vi "TSLIN_SetData.vi"(8 "Error in":errorcluster caption="error in (no error)", 9 "AppName":string="LABFD", 10 "Set":T1={"Hardware Type"=3, "Hardware Subtype"=enum."TC1026", "AHwChannel"=0, "AAppChannel"=0, "ABaudrateKbps"=19.2, "AProtocol"=2, "AldHW"=0} {"Hardware Type" items=["BUS_UNKNOWN_TYPE", "TS_TCP_DEVICE", "XL_USB_DEVICE", "TS_USB_DEVICE", "PEAK_USB_DEVICE", "KVASER_USB_DEVICE", "ZLG_USB_DEVICE", "ICS_USB_DEVICE", "TS_TC1005_DEVICE", "CANABLE_USB_DEVICE", "TS_WIRELESS_OBD", "TS_USB_DEVICE_EX", "IXXAT_USB_DEVICE", "TS_ETH_IF_DEVICE", "TS_USB_IF_DEVICE", "BUS_DEV_TYPE_COUNT"]; "AHwChannel" items=["CHN1", "CHN2", "CHN3", "CHN4", "CHN5", "CHN6", "CHN7", "CHN8", "CHN9", "CHN10", "CHN11", "CHN12", "CHN13", "CHN14", "CHN15", "CHN16", "CHN17", "CHN18", "CHN19", "CHN20", "CHN21", "CHN22", "CHN23", "CHN24", "CHN25", "CHN26", "CHN27", "CHN28", "CHN29", "CHN30", "CHN31", "CHN32"]; "AAppChannel" items=["CHN1", "CHN2", "CHN3", "CHN4", "CHN5", "CHN6", "CHN7", "CHN8", "CHN9", "CHN10", "CHN11", "CHN12", "CHN13", "CHN14", "CHN15", "CHN16", "CHN17", "CHN18", "CHN19", "CHN20", "CHN21", "CHN22", "CHN23", "CHN24", "CHN25", "CHN26", "CHN27", "CHN28", "CHN29", "CHN30", "CHN31", "CHN32"]; "AProtocol" items=["Lin_Protocol_13", "Lin_Protocol_20", "Lin_Protocol_21", "Lin_Protocol_J2602"]}, 11 "Path":path) -> (0 "Error out":errorcluster caption="error out", 1 "mapping_return":i32, 2 "config_baud_return":i32, 3 "Path output":path)   [LabVIEW 2014]
doc: "tsapp_set_mapping_verbose ：\nFunction Introduction ：\nBefore using hardware devices, map the channels (CAN/CANFD/LIN) for the application program\n(i.e. binding) specifies the designated channel of the CAN device. This operation can also be performed on\nThe device management interface of TSMaster is completed, and this part of the operation is not required in the code.\nRegarding the channel mapping function, there are still unclear areas. Please refer to the document: TsMasterApi HardwareMap.pdf\nCall location ：\nCall this function to complete the hardware binding before the application connects to the CAN tool.\ninput parameter \nAppName: Application Name: The name of the application bound to this Map, which should be consistent with the name in initialized lib_tsmaster\nagreement\nAAppChannelType: Channel type: including APP_CAN, APP_LIN AAppChannel: Channel number of the application: This is the channel number used by the upper level program\nAHardwareName: Hardware name: such as TOSUN, Vector, etc., can also be left blank, mainly for the convenience of users to view\nAHardwareType: Hardware type: According to TLIBBusToolDeviceType, it includes all mainstream CANs currently on the market\nCard hardware Among them, the definition of tool enumeration types is as follows:\npublic enum TLIBBusToolDeviceType : int {\nBUS_UNKNOWN_TYPE = 0, TS_TCP_DEVICE = 1, XL_USB_DEVICE = 2, TS_USB_DEVICE = 3, PEAK_USB_DEVICE = 4, KVASER_USB_DEVICE = 5, ZLG_USB_DEVICE = 6, ICS_USB_DEVICE = 7, TS_TC1005_DEVICE = 8\n};\nAHardwareSubType: The sub devices under this device type, such as TS-USB-Device on the same star, are included below TC1001, TL1002, TC1011 and other series of products\nAHardwareIndex: Supports inserting multiple identical hardware devices simultaneously, such as inserting two TC1001 devices at the same time. This is used to select\nIs it the channel of device 1 or device 2\nAHardwareChannel: The channel for hardware devices, for example, TC1005 has 5 hardware channels, and this parameter is used to select the appropriate one\nCorresponding hardware channels\nAEnable Mapping: Is this mapping enabled? If set to false, the channel cannot be used。\nReturn value ：\n==0: Execution successful\nOther: Query error code\n\ntsapp_configure_baudrate_lin :\nFunction Introduction\nSet parameters such as baud rate for LIN channel\nCall location\nBefore connecting hardware devices, set the parameters of the channel first\ninput parameter \nAIdxChnq: Application Channel Number\nABaud rate Kbps: baud rate (kbps)\nAProtocol: baud rate (kbps)\nReturn value\n==0: Connection successful\nOther: Check for error codes"
uses:
  Typedef/TSLIN_SetData.ctl
  Utilities/Typedef/Hardware_Subtype.ctl
  All_Control/Typedef/Hardware Type.ctl
panel:
  # "Use N CAN channels and set N CAN channels"
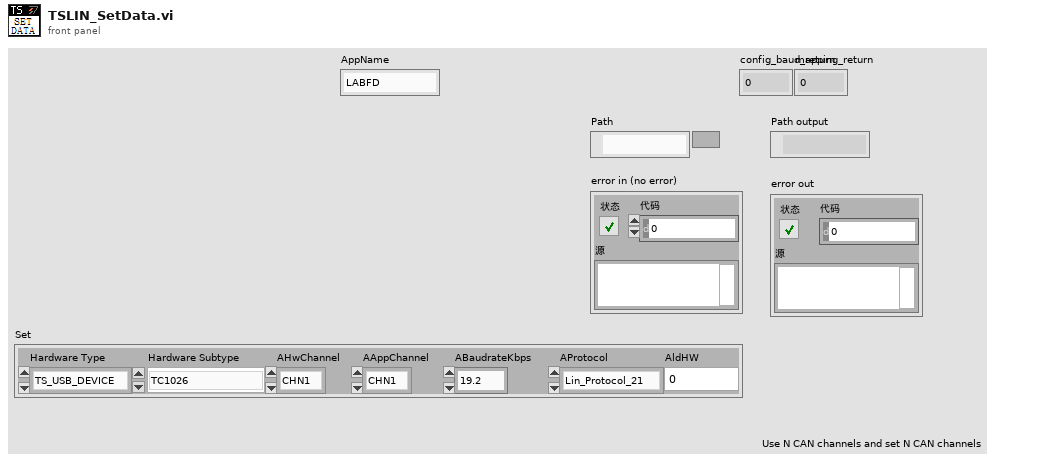
[diagram p1: front panel]
types:
  T1 = typedef "TSLIN_SetData.ctl" = cluster{"Hardware Type":T2, "Hardware Subtype":T3, "AHwChannel":i32, "AAppChannel":i32, "ABaudrateKbps":sgl, "AProtocol":i32, "AldHW":i32}
  T2 = typedef "Hardware Type.ctl" = i32
  T3 = typedef "Hardware_Subtype.ctl" = enum16{"TS_UNKNOWN_DEVICE", "TSCAN_PRO", "TSCAN_Lite1", "TC1001", "TL1001", "TC1011", "TM5011", "TC1002", "TC1014", "TSCANFD2517", "TC1026", "TC1016", "TC1012", "TC1013", "TLog1002", "TC1034", "TC1018", "GW2116", "TC2115", "MP1013", "TC1113", "TC1114", "TP1013", "TC1017", "TP1018", "TF10XX", "TL1004_FD_4_LIN_2", "TE1051", "TP1051", "TP1034", "TTS9015", "TP1026", "TTS1026", "TTS1034", "TTS1018", "TL1011", "TTS1015_LiAuto", "TTS1013_LiAuto", "TTS1016Pro", "TC1054Pro", "TC1054", "TLog1038", "TO1013", "TC1034Pro", "TC1018Pro", "TC1038Pro", "TS_DEV_END"}
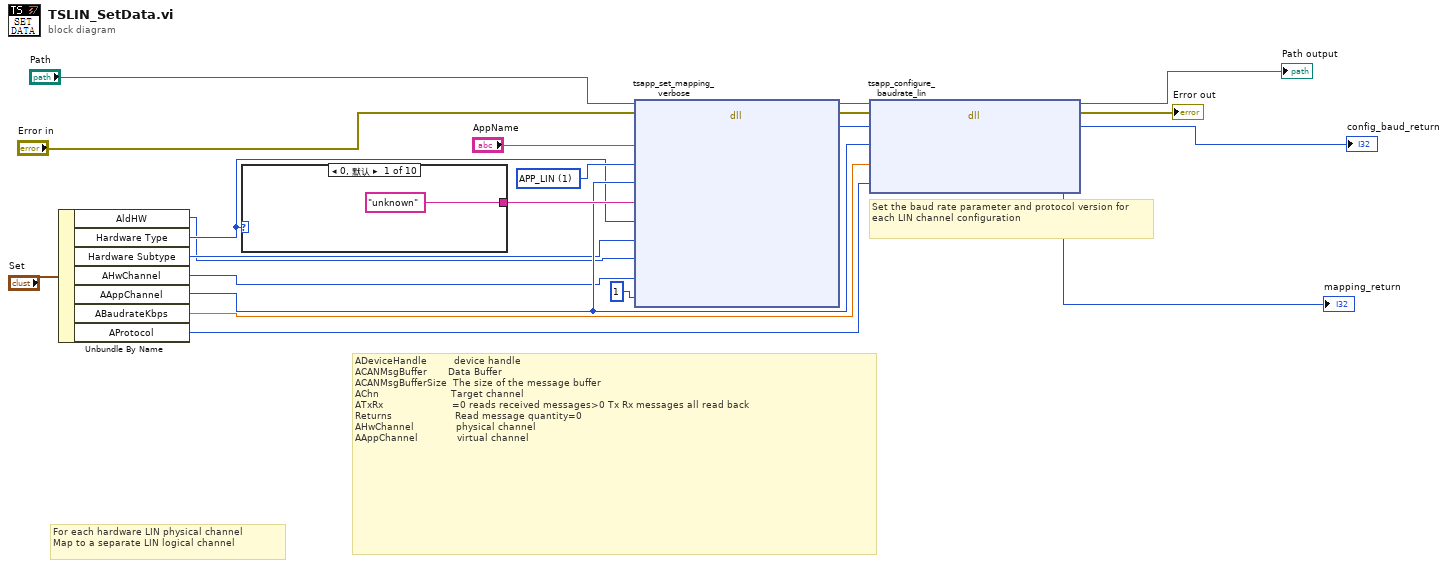
[diagram p0: block diagram]
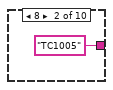
[diagram p2: hidden frame]
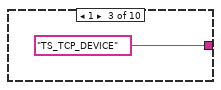
[diagram p3: hidden frame]
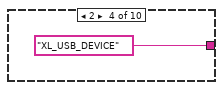
[diagram p4: hidden frame]
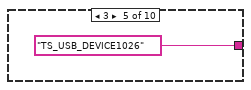
[diagram p5: hidden frame]
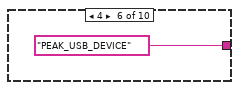
[diagram p6: hidden frame]
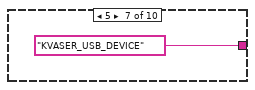
[diagram p7: hidden frame]
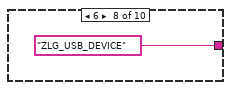
[diagram p8: hidden frame]
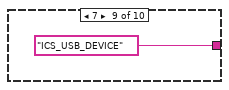
[diagram p9: hidden frame]
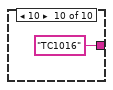
[diagram p10: hidden frame]
diagram:
  w19 = 1 items=["APP_CAN", "APP_LIN"] ("AAppChannelType")
  # "Set the baud rate parameter and protocol version for each LIN channel configuration"
  # "ADeviceHandle         device handle\nACANMsgBuffer       Data Buffer\nACANMsgBufferSize  The size of the message buffer\nAChn                        Target channel\nATxRx                       =0 reads received messages>0 Tx Rx messages all read back\nReturns                     Read message quantity=0\nAHwChannel              physical channel\nAAppChannel             virtual channel"
  # "For each hardware LIN physical channel\nMap to a separate LIN logical channel"
  n1 = Unbundle By Name("Set") -> ("AldHW"=w1:i32, "Hardware Type"=w7:T2, "Hardware Subtype"=w8:T3, "AHwChannel"=w2:i32, "AAppChannel"=w11:i32, "ABaudrateKbps"=w10:sgl, "AProtocol"=w9:i32)
  n2 = case shown="0, 默认" w7 {
    tunnel: ["unknown" ("AHardwareName") "TC1005" ("AHardwareName") "TS_TCP_DEVICE" ("AHardwareName") "XL_USB_DEVICE" ("AHardwareName") "TS_USB_DEVICE1026" ("AHardwareName") "PEAK_USB_DEVICE" ("AHardwareName") "KVASER_USB_DEVICE" ("AHardwareName") "ZLG_USB_DEVICE" ("AHardwareName") "ICS_USB_DEVICE" ("AHardwareName") "TC1016" ("AHardwareName")] -> w18
    frame 0, Default {
    }
    frame 8 {
    }
    frame 1 {
    }
    frame 2 {
    }
    frame 3 {
    }
    frame 4 {
    }
    frame 5 {
    }
    frame 6 {
    }
    frame 7 {
    }
    frame 10 {
    }
  }
  n3 = dll-call lib="PTH2Habs CUsers\nAdministratorDesktopTS_Can通讯PathTSMaster.dll" fn="tsapp_set_mapping_verbose"(path in="Path", error in="Error in", "FAPppName"="AppName", "AChnType"=w19, "FAppChannelIndex"=w11, "AHWDeviceName"=w18, "AHWDeviceType"=w7, "AHWDeviceSubType"=w8, "AldHW"=w1, "AldHWChn"=w2, "FMappingDisabled"=u32 1) -> (path out=w20:path, error out=w16:errorcluster, "return"=→"mapping_return":i32)  [unwired: 10 in]
  n4 = dll-call lib="PTH2@abs EDemo同星TSCAN_V1.4_20220301ConfigTSMaster.dll" fn="tsapp_configure_baudrate_lin"(path in=w20, error in=w16, "ALdxChn"=w11, "ABaudrateKbps"=w10, "AProtocol"=w9) -> (path out=→"Path output":path, error out=→"Error out":errorcluster, "return"=→"config_baud_return":i32)  [unwired: 4 in]
